vi "SUB_ASK_YESNO_RETST.vi"(3 "Question:":string) -> (1 "yes/no":enum32{"No Selection", "Yes", "No", "None"}(ring))   [LabVIEW 2011]
doc: "This is an example of how to use the radio buttons control with the Value Changed event."
panel:
  in  "Answer:Is it Correct ?":T1(radio)=enum."Yes"
  # "請回答 正確 或 NG"
  # "依據待測物實際狀況.點選上面選項"
  # "重測"
  # "正確"
  # "NG"
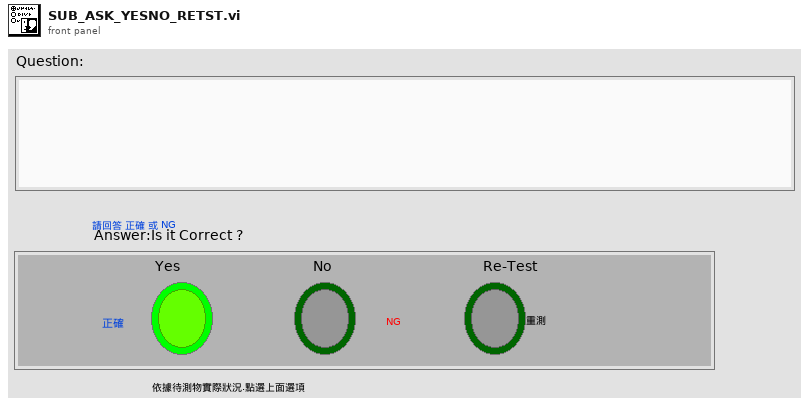
[diagram p1: front panel]
types:
  T1 = enum32{"No Selection", "Yes", "No", "None", "Re-Test"}
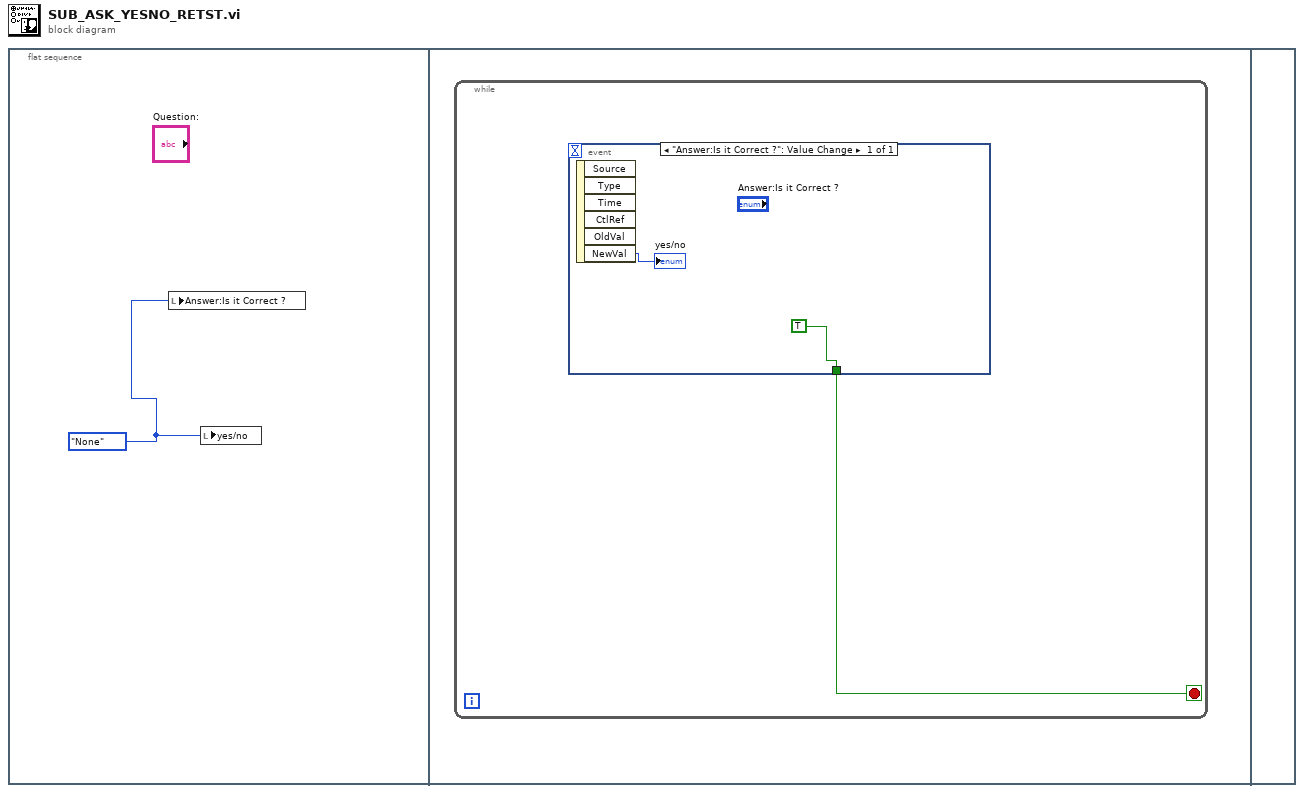
[diagram p0: block diagram]
diagram:
  n1 = flat-sequence {
    frame #0 {
      w1 = enum32{"No Selection", "Yes", "No", "None"}."None" ("yes/no")
      n2 = local write "Answer:Is it Correct ?"(w1) -> ()
      n3 = local write "yes/no"(w1) -> ()
    }
    frame #1 {
      n4 = while {
        stop <- w2 stop-if-true
        n5 = event shown="[0] \"Answer:Is it Correct ?\": Value Change" {
          selector: _ -> [_]
          dyn-events: _ -> [_]
          timeout: _ -> [_]
          tunnel: [TRUE] -> w2
          event "Answer:Is it Correct ?": Value Change {
            n6 = event-data() -> ("NewVal"=→"yes/no":T1)  [unwired: 1 in, 5 out]
          }
        }
      }
    }
    frame #2 {
    }
  }
